vi "TestParseWithUnknownFields.vi"() -> ()   [LabVIEW 2019]
uses:
  <vilib>/gRPC/LabVIEW gRPC Library/Server API/typeDefs/Any.ctl
  <vilib>/gRPC/LabVIEW gRPC Library/Server API/typeDefs/Message Metadata.ctl
  <vilib>/gRPC/LabVIEW gRPC Library/Server API/typeDefs/Message Element Metadata.ctl
  <vilib>/gRPC/LabVIEW gRPC Library/Server API/typeDefs/Message Element Type.ctl
  50cd6ca9-b915-40c5-a5da-5a0bdd109e0e.vi
  f62721b2-a209-4c6b-affd-5652a03b42cf.vi
  7d7811d0-96b0-480a-b9e1-7a69e0e26027.vi
  65d46b58-227a-49f8-b739-8ba8c807fa65.vi
  <vilib>/gRPC/LabVIEW gRPC Library/Server API/Server/Get Server DLL Path.vi
  <vilib>/gRPC/LabVIEW gRPC Library/gprc-lvsupport-release.lvlib
panel:
  out "error out":errorcluster
  out "Numeric 2":i32
  out "Any":T1
  out "Numeric":i32
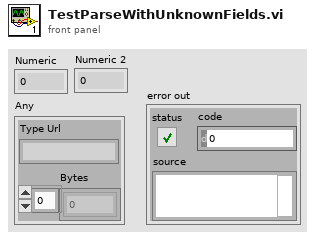
[diagram p1: front panel]
types:
  T1 = typedef "gprc-lvsupport-release.lvlib/Any.ctl" = cluster{"Type Url":string, "Bytes":u8[]}
  T2 = typedef "gprc-lvsupport-release.lvlib/Message Element Type.ctl" = enum32{"Int32Value", "FloatValue", "DoubleValue", "BoolValue", "StringValue", "MessageValue", "Int64Value", "UInt32Value", "UInt64Value", "EnumValue", "Bytes", "Fixed64", "Fixed32", "SFixed64", "SFixed32", "SInt64", "SInt32"}
  T3 = typedef "gprc-lvsupport-release.lvlib/Message Metadata.ctl" = cluster{"Version":i32, "Name":string, "Type Url":string, "Elements":T4[]}
  T4 = typedef "gprc-lvsupport-release.lvlib/Message Element Metadata.ctl" = cluster{"Embedded Message Name":string, "Protobuf Index":i32, "MessageElementType":T2, "Repeated":bool}
  T5 = typedef "gprc-lvsupport-release.lvlib/grpcId.ctl" = u64
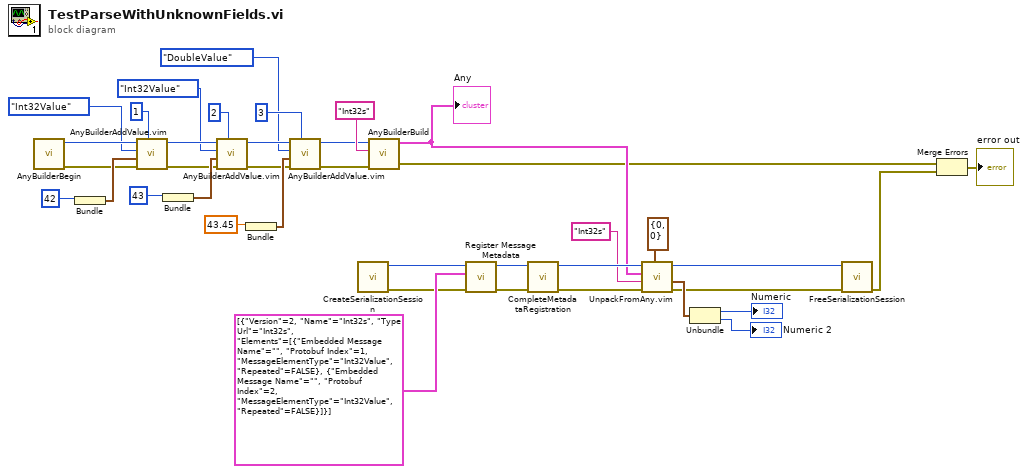
[diagram p0: block diagram]
diagram:
  n1 = call <vilib>:"AnyBuilderBegin.vi"() -> ("error out"=w11:errorcluster, "Builder Ref Out"=w39:T5)  [unwired: 9 in]
  n2 = Bundle(42) -> (w36:cluster{i32})  [unwired: 1 in]
  n3 = call "AnyBuilderAddValue.vim"("protobufId"=1, "error in (no error)"=w11, "Value"=w36, "MessageElementType"=Message_Element_Type."Int32Value", "gRPCid in"=w39) -> ("error out"=w10:errorcluster, "gRPCid"=w23:u64)  [unwired: 5 in]
  n4 = Bundle(43) -> (w19:cluster{i32})  [unwired: 1 in]
  n5 = call "AnyBuilderAddValue.vim"("protobufId"=2, "error in (no error)"=w10, "Value"=w19, "MessageElementType"=Message_Element_Type."Int32Value", "gRPCid in"=w23) -> ("error out"=w9:errorcluster, "gRPCid"=w17:u64)  [unwired: 5 in]
  n6 = Bundle(43.45) -> (w13:cluster{dbl})  [unwired: 1 in]
  n7 = call "AnyBuilderAddValue.vim"("protobufId"=3, "error in (no error)"=w9, "Value"=w13, "MessageElementType"=Message_Element_Type."DoubleValue", "gRPCid in"=w17) -> ("error out"=w8:errorcluster, "gRPCid"=w16:u64)  [unwired: 5 in]
  n8 = call <vilib>:"CreateSerializationSession.vi"() -> ("error out"=w7:errorcluster, "Serialization Session ID"=w34:T5)  [unwired: 10 in]
  n9 = call <vilib>:"AnyBuilderBuild.vi"("error in (no error)"=w8, "Message Type"="Int32s", "Builder Ref"=w16) -> ("error out"=w2:errorcluster, "Any"=w29:T1)  [unwired: 7 in]
  "Any" <- w29
  n10 = call <vilib>:"Register Message Metadata.vi"("error in (no error)"=w7, "Messages"=T3[] [{"Version"=2, "Name"="Int32s", "Type Url"="Int32s", "Elements"=[{"Embedded Message Name"="", "Protobuf Index"=1, "MessageElementType"=enum."Int32Value", "Repeated"=FALSE}, {"Embedded Message Name"="", "Protobuf Index"=2, "MessageElementType"=enum."Int32Value", "Repeated"=FALSE}]}], "gRPCid"=w34) -> ("error out"=w6:errorcluster, "gRPCid"=w31:T5)  [unwired: 7 in]
  n11 = call <vilib>:"CompleteMetadataRegistration.vi"("error in (no error)"=w6, "gRPC ID"=w31) -> ("error out"=w5:errorcluster, "gRPC ID Out"=w30:T5)  [unwired: 8 in]
  n12 = call "UnpackFromAny.vim"("Data Type"=cluster{i32, i32} {0, 0}, "error in (no error)"=w5, "Message Type"="Int32s", "Any"=w29, "gRPCid in"=w30) -> ("error out"=w4:errorcluster, "Unpacked Value"=w26:cluster{i32, i32}, "gRPCid"=w24:u64)  [unwired: 4 in]
  n13 = Unbundle(w26) -> (→"Numeric":i32, →"Numeric 2":i32)
  n14 = call <vilib>:"FreeSerializationSession.vi"("error in (no error)"=w4, "Serialization Session ID"=w24) -> ("error out"=w3:errorcluster)  [unwired: 9 in]
  n15 = Merge Errors(w2, w3) -> (→"error out":errorcluster)
